vi "Publish Image.vi"(8 "error in (no error)":errorcluster, 9 "Buffer Number":u32, 10 "Image":T1, 11 "IMAQdx Actor in":refnum<class "IMAQdx Actor.lvclass">) -> (0 "error out":errorcluster, 3 "IMAQdx Actor out":refnum<class "IMAQdx Actor.lvclass">)   [LabVIEW 2014, in "IMAQdx Actor.lvlib" / "IMAQdx Actor.lvclass"]
uses:
  IMAQdx Actor.lvclass
  <vilib>/vision/Image Controls.llb/IMAQ Image.ctl
  Camera Actor/Camera Actor/Camera Actor.lvclass/Camera Actor.ctl
  Camera Actor/Camera Actor Messages/New Image Msg/New Image Msg.lvclass/New Image Msg.ctl
  <vilib>/ActorFramework/Message Enqueuer/Message Enqueuer.lvclass/Message Enqueuer.ctl
  Camera Actor/Camera Actor/Read New Image Msg.vi
  Camera Actor/Camera Actor/Read Image Receiver.vi
  <vilib>/ActorFramework/Message Enqueuer/Enqueue.vi
  <vilib>/ActorFramework/Message Priority Queue/Priority Enqueue.vi
  Camera Actor/Camera Actor Messages/New Image Msg/New Image Msg.lvclass
  <vilib>/ActorFramework/Message Enqueuer/Message Enqueuer.lvclass
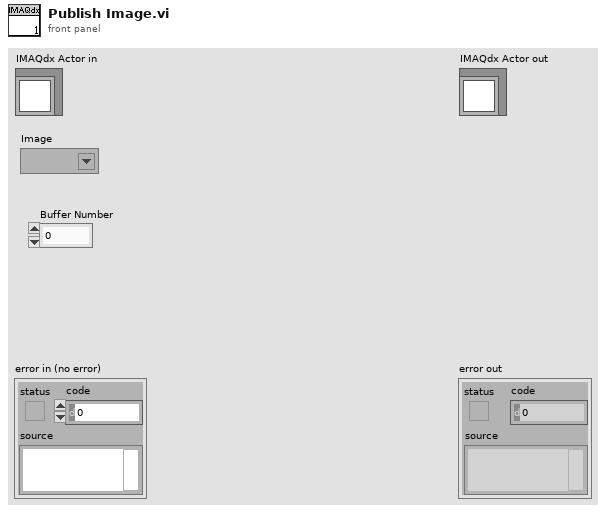
[diagram p1: front panel]
types:
  T1 = typedef "IMAQ Image.ctl" = refnum<image>
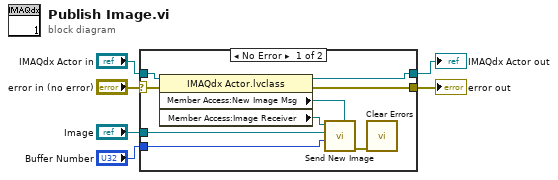
[diagram p0: block diagram]
diagram:
  n1 = case shown="No Error" "error in (no error)" {
    selector: "error in (no error)" -> [w8 w17]
    tunnel: [w7 w17] -> w5
    tunnel: [w11 w16] -> w3
    tunnel: "IMAQdx Actor in" -> [w15 w16]
    tunnel: "Image" -> [w13 _]
    tunnel: "Buffer Number" -> [w12 _]
    frame No Error {
      n2 = property class="IMAQdx Actor.lvclass"(reference=w15, error in=w8) -> (reference out=w11:refnum<class "IMAQdx Actor.lvclass">, error out=w7:errorcluster, "Member Access:New Image Msg"=w10:refnum<class "New Image Msg.lvclass">, "Member Access:Image Receiver"=w9:refnum<class "Message Enqueuer.lvclass">)
      n3 = call "Send New Image.vi"("Message Type"=w10, "Buffer Number"=w12, "Image"=w13, "Message Enqueuer"=w9) -> ("error out"=w14:errorcluster)  [unwired: 6 in, 1 out]
      n4 = call <vilib>:"Clear Errors.vi"("error in (no error)"=w14) -> ()  [unwired: 5 in, 2 out]
    }
    frame Error {
    }
  }
  "error out" <- w5
  "IMAQdx Actor out" <- w3
